vi "resonant.scan.engine_rrMD.vi"() -> ()   [LabVIEW 2012]
doc: "SciScan 1.2 160622"
uses:
  <vilib>/Utility/VariantDataType/Type.ctl
  hyperscope modules/hyperscope subVIs/Timebase and Trigger Routing.ctl
  GFG/GFGnumericGet.vi
  GFG/GFGbooleanGet.vi
  GFG/GFGstringGet.vi
  <vilib>/Utility/error.llb/Error Cluster From Error Code.vi
  <vilib>/rvi/errors/niLvFpgaAdjustHostInterfaceError.vi
  GFG/GFGfpRefGet.vi
  <vilib>/FPGAPlugInAG/Dynamic/niLvFpga_Abort_Dynamic.vi
  <vilib>/FPGAPlugInAG/Dynamic/niLvFpga_Close_Dynamic.vi
  <vilib>/rvi/interface/nirviReadWriteControl/nirviReadWriteControl.xnode
  Custom Controls/FPGA reference typedef for 120MHz code.ctl
  <vilib>/rvi/interface/nirviMethod/nirviMethod.xnode
  <vilib>/rvi/interface/nirviCloseFPGA/nirviCloseFPGA.xnode
  GFG/GFG library.lvlib
  <vilib>/Utility/VariantDataType/VariantType.lvlib
  NiFpgaLv.dll
  <vilib>/rvi/interface/Simulation/niFpgaSimulationCallBeginRW.vi
  <vilib>/FPGAPlugInAG/Dynamic/niLvFpga_ReadFifo_Dynamic.vi
  <vilib>/rvi/errors/niLvFpgaMergeErrorWithErrorCode.vi
panel:
  out "error out 2":errorcluster
  out "error out":errorcluster
  out "x/y":dbl format="%#_6f"
  out "max Elements Remaining":u32
  out "size(s)":i32[](array[numeric])
  out "Elements Remaining":u32
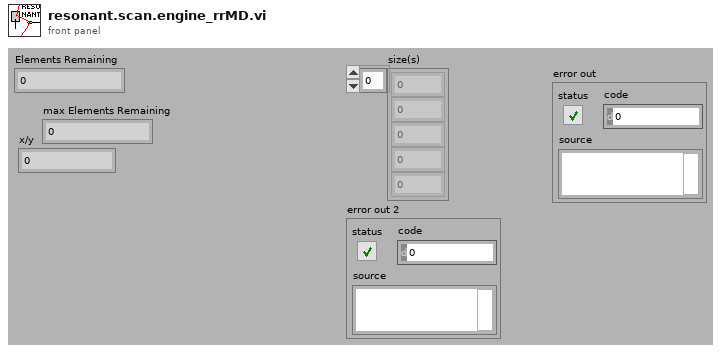
[diagram p1: front panel]
types:
  T1 = typedef "Timebase and Trigger Routing.ctl" = enum16{"Connect", "Disconnect all", "Disconnect Trigger"}
  T2 = enum8{"Enabled", "Disabled", "Disabled and Grayed Out"}
  T3 = typedef "biotfile select.ctl" = enum16{"7962with5751_512px_40Mhz", "7962with5751_512px_50Mhz", "7961with5734_1024px_120Mhz or ext lasersync", "7962with5734_1024px_120Mhz or ext lasersync", "7962with5734_512px_120Mhz or ext lasersync", "7961with5734_512px_120Mhz or ext lasersync", "7962with5751_12kHz_512px_50MHz_4ch", "7962with5751_1536px_2ch_40Mhz", "7962with5751_1536px_2ch_50Mhz", "7962with5751_12kHz_1024px_2ch_50MHz"}
  T4 = typedef "FPGA reference typedef for 120MHz code.ctl" = refnum<k20>
  T5 = cluster{"[0]":bool, "[1]":bool, "[2]":bool, "[3]":bool, "[4]":bool, "[5]":bool, "[6]":bool, "[7]":bool, "[8]":bool}
  T6 = cluster{cluster{"[0]":bool, "[1]":bool, "[2]":bool, "[3]":bool, "[4]":bool, "[5]":bool, "[6]":bool, "[7]":bool, "[8]":bool}, cluster{"[0]":bool, "[1]":bool, "[2]":bool, "[3]":bool, "[4]":bool, "[5]":bool, "[6]":bool, "[7]":bool, "[8]":bool}}
  T7 = cluster{"WaveformChartRef":refnum<vi>, "DigitalRef":refnum<vi>, "ArrayRef":refnum<vi>, "TabControlRef":refnum<vi>, "EnumRef":refnum<vi>, "RingRef":refnum<vi>, "BooleanRef":refnum<vi>, "KnobRef":refnum<vi>, "SlideRef":refnum<vi>, "PathRef":refnum<vi>, "StringRef":refnum<vi>, "ComboBox":refnum<vi>, "WaveformGraphRef":refnum<vi>}
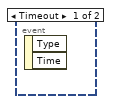
[diagram p5: hidden frame]
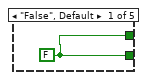
[diagram p6: hidden frame]
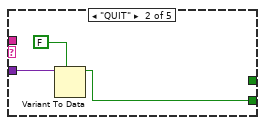
[diagram p7: hidden frame]
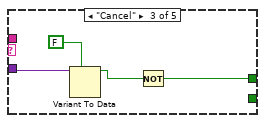
[diagram p8: hidden frame]
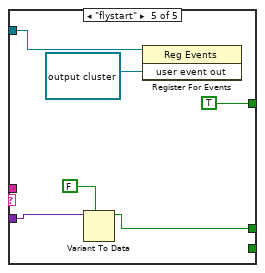
[diagram p10: hidden frame]
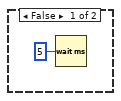
[diagram p11: hidden frame]
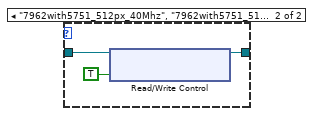
[diagram p12: hidden frame]
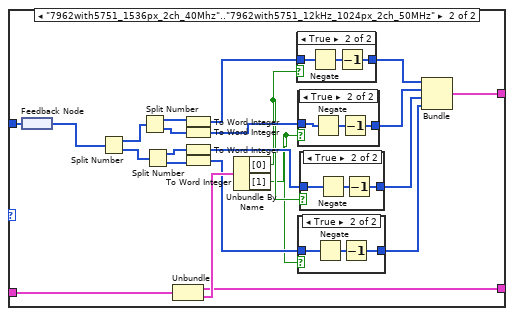
[diagram p20: hidden frame]
diagram:
  n1 = call "GFG_core.vi"() -> ("user event out"=w2:refnum<user-event>)  [unwired: 13 in, 6 out]
  n2 = register-events(w2) -> (reference out=w3:refnum<event-registration>)  [unwired: 2 in, 1 out]
  n3 = while {
    shift-right: [w4] -> _
    shift-left: w3 -> [w11]
    tunnel: w2 -> [w10]
    border: u32 1000000 ("Elements Remaining") -> [_]
    stop <- w12 stop-if-true
    n4 = event shown="[1] <user event out>: User Event" {
      selector: w11 -> [_ w32]
      dyn-events: [_ _] -> w8
      timeout: _ -> [_ _]
      tunnel: [_ w36] -> w13
      tunnel: [_ w35] -> w12
      tunnel: [_ w31] -> w7
      tunnel: [_ w30] -> w6
      event Timeout {
        n5 = event-data() -> ()  [unwired: 1 in, 2 out]
      }
      event User Event {
        n6 = event-data() -> ("Source VI"=w33:string, "Variable Name"=w30:string, "Variant"=w34:variant)  [unwired: 1 in, 4 out]
        n7 = case shown="\"FOCUS\", \"Record\"" w30 {
          tunnel: [w37 _ w41 w49 w54] -> w36
          tunnel: [w37 w38 _ _ _] -> w35
          tunnel: w34 -> [_ w40 w43 w50 w58]
          tunnel: w33 -> [_ _ _ w48 _]
          tunnel: w32 -> [_ _ _ w46 w55]
          tunnel: [_ _ _ TRUE TRUE] -> w31
          frame "False", Default {
            w37 = FALSE ("NewVal")
          }
          frame "QUIT" {
            n8 = Variant To Data(type=FALSE ("NewVal"), Variant=w40) -> (data=w38:bool)  [unwired: 1 in, 1 out]
          }
          frame "Cancel" {
            n9 = Variant To Data(type=FALSE ("NewVal"), Variant=w43) -> (data=w42:bool)  [unwired: 1 in, 1 out]
            n10 = Not(x=w42) -> (.not. x?=w41:bool)
          }
          frame "FOCUS", "Record" {
            n11 = case shown="\"fp button handler_crMD.vi\"" w48 {
              tunnel: w50 -> [_ w52]
              tunnel: [_ w51] -> w49
              frame "False", Default {
              }
              frame "fp button handler_crMD.vi" {
                n12 = Variant To Data(type=FALSE ("NewVal"), Variant=w52) -> (data=w51:bool)  [unwired: 1 in, 1 out]
              }
            }
            n13 = register-events(reference=w46, refnum<user-event> refnum ("user event out")) -> ()  [unwired: 1 in, 2 out]
          }
          frame "flystart" {
            n14 = Variant To Data(type=FALSE ("NewVal"), Variant=w58) -> (data=w54:bool)  [unwired: 1 in, 1 out]
            n15 = register-events(reference=w55, refnum<user-event> refnum ("user event out")) -> ()  [unwired: 1 in, 2 out]
          }
        }
      }
    }
    n16 = case shown="True" w13 {
      tunnel: [_ w120] -> w9
      tunnel: w6 -> [_ w102]
      tunnel: [_ w112] -> w5
      frame False {
        n17 = Wait (ms)(milliseconds to wait=u32 5) -> ()  [unwired: 1 out]
      }
      frame True {
        (unwired) FALSE
        w80 = u64[] [] ("Data")
        n18 = call "GFG_core.vi"("Variable Name in"="flystart" ("Tag in"), "Variant in"=FALSE, "Action"=enum16{"Init", "Set", "Get"}."Set") -> ("error out"=w113:errorcluster)  [unwired: 10 in, 6 out]
        n19 = flat-sequence {
          tunnel: w102 -> [w192]
          tunnel: [w192] -> w61
          tunnel: [w198] -> w101
          tunnel: w61 -> [w198]
          frame #0 {
            n20 = call "GFG_core.vi"("Variable Name in"="scanengine_running", "Variant in"=TRUE, "Action"=enum16{"Init", "Set", "Get"}."Set") -> ()  [unwired: 10 in, 7 out]
          }
          frame #1 {
            n21 = call "GFG_core.vi"("Variable Name in"="flystop", "Variant in"=FALSE ("Boolean"), "Action"=enum16{"Init", "Set", "Get"}."Set") -> ()  [unwired: 10 in, 7 out]
            n22 = call "disable fp elements during scanning.vi"("T for grey out"=TRUE) -> ()  [unwired: 11 in]
            n23 = call "GFG_core.vi"("Variable Name in"="display every n-th frame" ("Tag in"), "Variant in"=2.0 ("Numeric"), "Action"=enum16{"Init", "Set", "Get"}."Set") -> ()  [unwired: 10 in, 7 out]
          }
        }
        n24 = call-poly "GFGpolyGet.vi"("Variable Name in"="frames.p.queue.item" ("Tag in")) -> ("Numeric"=w107:dbl)  [unwired: 8 in, 2 out]
        n25 = call-poly "GFGpolyGet.vi"("error in (no error)"=w113, "Variable Name in"="no..of.frames.to.acquire" ("Tag in")) -> ("Numeric"=w106:dbl)  [unwired: 7 in, 2 out]
        n26 = Divide(x=w106, y=w107) -> (x/y=w108:dbl)
        n27 = flat-sequence {
          tunnel: w94 -> [w150]
          tunnel: w93 -> [w149]
          tunnel: w77 -> [_]
          tunnel: [errorcluster {"status"=FALSE, "code"=0, "source"=""} ("error out")] -> w76
          tunnel: [w153] -> w75
          tunnel: [w152] -> w74
          tunnel: [w151] -> w73
          tunnel: [w148] -> w72
          tunnel: w76 -> [w162]
          tunnel: w75 -> [w161]
          tunnel: w74 -> [w160]
          tunnel: w73 -> [w159]
          tunnel: w72 -> [w158]
          tunnel: [w162] -> w69
          tunnel: [w161] -> w68
          tunnel: [w160] -> w67
          tunnel: [w159] -> w66
          tunnel: [w158] -> w65
          tunnel: [w164] -> w70
          tunnel: [w165] -> w82
          tunnel: [w166] -> w79
          tunnel: [w167] -> w71
          tunnel: [w168] -> w64
          tunnel: w69 -> [w168]
          tunnel: w68 -> [w167]
          tunnel: w67 -> [w166]
          tunnel: w66 -> [w165]
          tunnel: w65 -> [w164]
          frame #0 {
            n28 = call-poly "GFGpolyGet.vi"("Variable Name in"="Hyperscope") -> ("Boolean Value OUT"=w143:bool)  [unwired: 9 in, 1 out]
            n29 = case shown="True" w143 {
              frame False {
              }
              frame True {
                n30 = call-poly "GFGpolyGet.vi"("Variable Name in"="scanner.type") -> ("String"=w146:string)  [unwired: 9 in, 1 out]
                n31 = call "Timebase and Trigger Routing.vi"("Signal Router Action"=Timebase_and_Trigger_Routing."Connect", "System Type"=w146) -> ()  [unwired: 9 in, 1 out]
              }
            }
          }
          frame #1 {
            n32 = call "configure resonance.vi"("x resonant zoom voltage"=w149, "Start Delay (Ticks)"=w150) -> ("bitfile name"=w148:T3, "pixels per frame"=w152:dbl, "FPGA VI Reference Out"=w153:T4, "Actual Depth 3"=w151:u32)  [unwired: 6 in]
          }
          frame #2 {
            n33 = call "GFG_core.vi"("Variable Name in"="shutter" ("Tag in"), "Variant in"=TRUE, "Action"=enum16{"Init", "Set", "Get"}."Set") -> ()  [unwired: 10 in, 7 out]
          }
          frame #3 {
            n34 = Wait (ms)(milliseconds to wait=u32 20) -> ()  [unwired: 1 out]
          }
        }
        n35 = Increment(x=w108) -> (x+1=w103:dbl)
        n36 = call "check focus or flystart.vi"("GFG variable name"=w101) -> ("Focus or flystart?"=w77:bool)  [unwired: 10 in]
        n37 = Round Toward +Infinity(x=w103) -> (ceil(x): smallest int >= x=w105:dbl)
        n38 = Select(t=inf, s=w77, f=w105) -> (s? t:f=w117:dbl)
        n39 = call-poly "GFGpolyGet.vi"("Variable Name in"="Start.Delay" ("Tag in")) -> ("Numeric"=w94:dbl)  [unwired: 8 in, 2 out]
        n40 = call-poly "GFGpolyGet.vi"("Variable Name in"="x.voltage" ("Tag in")) -> ("Numeric"=w93:dbl)  [unwired: 8 in, 2 out]
        n41 = for {
          N: 4 -> [_]
          tunnel: "save.ch." ("Tag in") -> [w175]
          tunnel: [w173] -> w88 mode=indexing
          tunnel: "invert.ch." ("Tag in") -> [w171]
          tunnel: [w169] -> w87 mode=indexing
          i -> [w177]
          n42 = Increment(x=w177) -> (x+1=w176:i32)
          n43 = Number To Decimal String(number=w176) -> (decimal integer string=w170:string)  [unwired: 1 in]
          n44 = Concatenate Strings(w175, w170) -> (w174:string)
          n45 = Concatenate Strings(w171, w170) -> (w172:string)
          n46 = call-poly "GFGpolyGet.vi"("Variable Name in"=w174) -> ("Boolean Value OUT"=w173:bool)  [unwired: 9 in, 1 out]
          n47 = call-poly "GFGpolyGet.vi"("Variable Name in"=w172) -> ("Boolean Value OUT"=w169:bool)  [unwired: 9 in, 1 out]
        }
        n48 = Array To Cluster(array=w88) -> (cluster=w86:T5)
        n49 = Array To Cluster(array=w87) -> (cluster=w85:T5)
        n50 = Boolean To (0,1)(Boolean=w88) -> (0, 1=w91:i16[])
        n51 = Bundle(w86, w85) -> (w84:T6)  [unwired: 1 in]
        n52 = Add Array Elements(numeric array=w91) -> (sum=w90:i16)
        n53 = case shown="Default" w70 {
          tunnel: [w135 w138] -> w63
          tunnel: w71 -> [w134 w137]
          frame Default {
            n54 = xnode "Read/Write Control"("FPGA VI Reference In"=w134, "stop IO config loop"=TRUE, "stop IO config loop"=FALSE) -> ("FPGA VI Reference Out"=w135:T4)  [unwired: 1 in, 1 out]
          }
          frame "7962with5751_512px_40Mhz", "7962with5751_512px_50Mhz", "7962with5751_12kHz_512px_50MHz_4ch".."7962with5751_12kHz_1024px_2ch_50MHz" {
            n55 = xnode "Read/Write Control"("FPGA VI Reference In"=w137, "stop IO config loop"=TRUE) -> ("FPGA VI Reference Out"=w138:T4)  [unwired: 1 in, 1 out]
          }
        }
        n56 = case shown="\"7962with5751_1536px_2ch_40Mhz\"..\"7962with5751_12kHz_1024px_2ch_50MHz\"" w70 {
          tunnel: w79 -> [w139 w141]
          tunnel: [w139 w140] -> w78
          frame Default {
          }
          frame "7962with5751_1536px_2ch_40Mhz".."7962with5751_12kHz_1024px_2ch_50MHz" {
            n57 = Divide(x=w141, y=2.0) -> (x/y=w140:dbl)
          }
        }
        n58 = Initialize Array(i16 0, w107, w90, w79) -> (w81:i16[][][])
        n59 = Obtain Queue(name (unnamed)="resonance raw queue", element data type=w81) -> (queue out=w62:refnum<queue>)  [unwired: 3 in, 2 out]
        n60 = Tick Count (ms)() -> (millisecond timer value=w100:u32)
        n61 = flat-sequence {
          tunnel: w64 -> [_]
          tunnel: w63 -> [w131]
          tunnel: w62 -> [w130]
          frame #0 {
            n62 = call "external trigger warning resonant.vi"("queue ref in"=w130, "FPGA VI Reference In"=w131) -> ()  [unwired: 10 in]
          }
        }
        n63 = while {
          tunnel: [w234] -> w110
          tunnel: w62 -> [w237]
          tunnel: [w236] -> w129
          tunnel: w117 -> [w235]
          tunnel: w64 -> [w228]
          tunnel: w63 -> [w214]
          tunnel: w78 -> [w229]
          tunnel: [w227] -> w124
          tunnel: [w226] -> w122
          tunnel: w77 -> [w207]
          tunnel: w106 -> [w225]
          tunnel: [w202] -> w112
          shift-right: [w203] -> _
          shift-left: w81 -> [w230]
          tunnel: w107 -> [w211]
          tunnel: w107 -> [_]
          border: 0 ("x+y") -> [_]
          tunnel: w82 -> [w218]
          shift-right: [w215] -> _
          shift-left: 0 ("x+y") -> [w216]
          border: w100 -> [_]
          tunnel: w84 -> [w213]
          tunnel: w70 -> [w205]
          border: w80 -> [_]
          border: w80 -> [_]
          i -> [w209]
          stop <- w202 stop-if-true
          n64 = Equal To 0?(x=w209) -> (x = 0?=w201:bool)
          n65 = Increment(x=w209) -> (x+1=w212:i32)
          n66 = Increment(x=w211) -> (x+1=w204:dbl)
          n67 = Select(t=w204, s=w201, f=w211) -> (s? t:f=w210:dbl)
          n68 = case shown="True" w201 {
            frame False {
            }
            frame True {
              n69 = Build Array("Start.Delay" ("Variable Name in"), "ZOOM" ("Variable Name in"), "x.correction" ("Variable Name in")) -> (w238:string[])
              n70 = for {
                tunnel: w238 -> [w242] mode=indexing
                n71 = call-poly "GFGpolyGet.vi"("Variable Name in"=w242) -> ("output cluster"=w245:T7)  [unwired: 9 in, 1 out]
                n72 = Unbundle By Name(w245) -> ("SlideRef"=w243:refnum<vi>)
                n73 = property class="Slide"(reference=w243, "DisabledEnum"=T2."Enabled" ("Disabled")) -> ()  [unwired: 1 in, 2 out]
              }
            }
          }
          n74 = for {
            N: w210 -> [_]
            tunnel: [w283] -> w219
            tunnel: w228 -> [w283]
            tunnel: w229 -> [w253]
            tunnel: w214 -> [w282]
            shift-right: [w280] -> w203
            shift-left: w230 -> [w281]
            tunnel: w211 -> [w279]
            tunnel: w201 -> [w278]
            tunnel: w218 -> [w277]
            shift-right: [w275] -> w215
            shift-left: w216 -> [w276]
            tunnel: w209 -> [w274]
            tunnel: w213 -> [w271]
            tunnel: w201 -> [w270]
            tunnel: w205 -> [w247]
            i -> [w269]
            n75 = xnode "Invoke Method"("FPGA VI Reference In"=w282, "Number of Elements"=w253, "Timeout (ms)"=-1) -> ("error out"=→"error out 2":errorcluster, "Data"=w273:u64[], "Elements Remaining"=w254:u32)  [unwired: 1 in, 1 out]
            "Elements Remaining" <- w254
            n76 = case shown="Default" w247 {
              tunnel: w273 -> [w307 w345]
              tunnel: w271 -> [w306 w344]
              tunnel: [w285 w327] -> w251
              tunnel: [w284 w326] -> w250
              frame Default {
                n77 = feedback #1() -> (w303:u64[])
                n78 = feedback-in #1(w307) -> ()
                n79 = Split Number(x=w303) -> (hi(x)=w304:u32[], lo(x)=w305:u32[])
                n80 = Split Number(x=w304) -> (hi(x)=w301:u16[], lo(x)=w302:u16[])
                n81 = Split Number(x=w305) -> (hi(x)=w300:u16[], lo(x)=w299:u16[])
                n82 = Unbundle(w306) -> (w284:T5, w298:T5)
                n83 = To Word Integer(number=w301) -> (16bit integer=w290:i16[])
                n84 = To Word Integer(number=w302) -> (16bit integer=w292:i16[])
                n85 = To Word Integer(number=w300) -> (16bit integer=w293:i16[])
                n86 = To Word Integer(number=w299) -> (16bit integer=w291:i16[])
                n87 = Unbundle By Name(w298) -> ("[0]"=w297:bool, "[1]"=w296:bool, "[2]"=w295:bool, "[3]"=w294:bool)
                n88 = case shown="True" w297 {
                  tunnel: [w320 w321] -> w289
                  tunnel: w290 -> [w320 w323]
                  frame False {
                  }
                  frame True {
                    n89 = Negate(x=w323) -> (-x=w322:i16[])
                    n90 = Decrement(x=w322) -> (x-1=w321:i16[])
                  }
                }
                n91 = case shown="True" w296 {
                  tunnel: [w316 w317] -> w288
                  tunnel: w292 -> [w316 w319]
                  frame False {
                  }
                  frame True {
                    n92 = Negate(x=w319) -> (-x=w318:i16[])
                    n93 = Decrement(x=w318) -> (x-1=w317:i16[])
                  }
                }
                n94 = case shown="True" w294 {
                  tunnel: [w308 w309] -> w286
                  tunnel: w291 -> [w308 w311]
                  frame False {
                  }
                  frame True {
                    n95 = Negate(x=w311) -> (-x=w310:i16[])
                    n96 = Decrement(x=w310) -> (x-1=w309:i16[])
                  }
                }
                n97 = case shown="True" w295 {
                  tunnel: [w312 w313] -> w287
                  tunnel: w293 -> [w312 w315]
                  frame False {
                  }
                  frame True {
                    n98 = Negate(x=w315) -> (-x=w314:i16[])
                    n99 = Decrement(x=w314) -> (x-1=w313:i16[])
                  }
                }
                n100 = Bundle(w289, w288, w287, w286) -> (w285:cluster{i16[], i16[], i16[], i16[]})  [unwired: 1 in]
              }
              frame "7962with5751_1536px_2ch_40Mhz".."7962with5751_12kHz_1024px_2ch_50MHz" {
                n101 = feedback #2() -> (w341:u64[])
                n102 = feedback-in #2(w345) -> ()
                n103 = Split Number(x=w341) -> (hi(x)=w342:u32[], lo(x)=w343:u32[])
                n104 = Split Number(x=w342) -> (hi(x)=w339:u16[], lo(x)=w340:u16[])
                n105 = Split Number(x=w343) -> (hi(x)=w338:u16[], lo(x)=w337:u16[])
                n106 = Unbundle(w344) -> (w326:T5, w336:T5)
                n107 = To Word Integer(number=w339) -> (16bit integer=w332:i16[])
                n108 = To Word Integer(number=w340) -> (16bit integer=w334:i16[])
                n109 = To Word Integer(number=w338) -> (16bit integer=w335:i16[])
                n110 = To Word Integer(number=w337) -> (16bit integer=w333:i16[])
                n111 = Unbundle By Name(w336) -> ("[0]"=w325:bool, "[1]"=w324:bool)
                n112 = case shown="True" w325 {
                  tunnel: [w358 w359] -> w331
                  tunnel: w332 -> [w358 w361]
                  frame False {
                  }
                  frame True {
                    n113 = Negate(x=w361) -> (-x=w360:i16[])
                    n114 = Decrement(x=w360) -> (x-1=w359:i16[])
                  }
                }
                n115 = case shown="True" w324 {
                  tunnel: [w354 w355] -> w330
                  tunnel: w334 -> [w354 w357]
                  frame False {
                  }
                  frame True {
                    n116 = Negate(x=w357) -> (-x=w356:i16[])
                    n117 = Decrement(x=w356) -> (x-1=w355:i16[])
                  }
                }
                n118 = case shown="True" w324 {
                  tunnel: [w346 w347] -> w328
                  tunnel: w333 -> [w346 w349]
                  frame False {
                  }
                  frame True {
                    n119 = Negate(x=w349) -> (-x=w348:i16[])
                    n120 = Decrement(x=w348) -> (x-1=w347:i16[])
                  }
                }
                n121 = case shown="True" w325 {
                  tunnel: [w350 w351] -> w329
                  tunnel: w335 -> [w350 w353]
                  frame False {
                  }
                  frame True {
                    n122 = Negate(x=w353) -> (-x=w352:i16[])
                    n123 = Decrement(x=w352) -> (x-1=w351:i16[])
                  }
                }
                n124 = Bundle(w331, w330, w329, w328) -> (w327:cluster{i16[], i16[], i16[], i16[]})  [unwired: 1 in]
              }
            }
            n125 = feedback #3() -> (w260:u32)
            n126 = Greater?(x=w254, y=w260) -> (0:w262:bool)
            n127 = Or(x=w262, y=w278) -> (x .or. y?=w259:bool)
            n128 = feedback #4() -> (w248:u32)  [unwired: 1 in]
            n129 = case shown="True" w259 {
              tunnel: w254 -> [_ w460]
              tunnel: [w452 w460] -> w261
              tunnel: w260 -> [w452 _]
              tunnel: w277 -> [_ w459]
              tunnel: [w451 u32 1 ("x")] -> w249
              tunnel: w248 -> [w450 _]
              frame False {
                n130 = Increment(x=w450) -> (x+1=w451:u32)
              }
              frame True {
                n131 = Divide(x=w460, y=w459) -> (x/y=w458:dbl)
                n132 = Multiply(x=w458, y=100.0) -> (x*y=w455:dbl)
                "x/y" <- w455
                n133 = Greater?(x=w455, y=10.0) -> (0:w456:bool)
                n134 = case shown="True" w456 {
                  frame False {
                  }
                  frame True {
                    w463 = "display every n-th frame" ("Tag in")
                    n135 = call-poly "GFGpolyGet.vi"("Variable Name in"=w463) -> ("Numeric"=w462:dbl)  [unwired: 8 in, 2 out]
                    n136 = Increment(x=w462) -> (x+1=w461:dbl)
                    n137 = call "GFG_core.vi"("Variable Name in"=w463, "Variant in"=w461, "Action"=enum16{"Init", "Set", "Get"}."Set") -> ()  [unwired: 10 in, 7 out]
                  }
                }
                "max Elements Remaining" <- w460
              }
            }
            n138 = feedback-in #3(w261) -> ()
            n139 = feedback-in #4(w249) -> ()
            n140 = Less Or Equal?(x=w269, y=0) -> (x <= y?=w256:bool)
            n141 = And(x=w270, y=w256) -> (x .and. y?=w252:bool)
            n142 = Increment(x=w276) -> (x+1=w275:i32)
            n143 = case shown="False" w252 {
              tunnel: w281 -> [w370 w449]
              tunnel: [w369 w449] -> w280
              tunnel: w269 -> [w367 _]
              tunnel: w270 -> [w368 _]
              tunnel: w247 -> [w365 _]
              tunnel: w251 -> [w363 _]
              tunnel: w250 -> [w362 _]
              frame False {
                n144 = Decrement(x=w367) -> (x-1=w364:i32)
                n145 = Select(t=w364, s=w368, f=w367) -> (s? t:f=w366:i32)
                n146 = case shown="\"7962with5751_1536px_2ch_40Mhz\"..\"7962with5751_12kHz_1024px_2ch_50MHz\"" w365 {
                  tunnel: w370 -> [w385 w418]
                  tunnel: [w379 w415] -> w369
                  tunnel: w366 -> [w382 w410]
                  tunnel: w363 -> [w378 w409]
                  tunnel: w362 -> [w373 w404]
                  frame "7962with5751_1536px_2ch_40Mhz".."7962with5751_12kHz_1024px_2ch_50MHz" {
                    n147 = Unbundle(w378) -> (w377:i16[], w374:i16[], w376:i16[], w375:i16[])
                    n148 = Unbundle By Name(w373) -> ("[0]"=w372:bool, "[1]"=w371:bool)
                    n149 = Interleave 1D Arrays(w377, w376) -> (w381:i16[])
                    n150 = Interleave 1D Arrays(w374, w375) -> (w380:i16[])
                    n151 = case shown="True" w372 {
                      tunnel: w385 -> [w393 w399]
                      tunnel: [w393 w398] -> w384
                      tunnel: w382 -> [_ w397]
                      tunnel: w381 -> [_ w396]
                      tunnel: [0 w394] -> w383
                      frame False {
                      }
                      frame True {
                        w395 = 0 ("disabled index (row)")
                        n152 = Increment(x=w395) -> (x+1=w394:i32)
                        n153 = Replace Array Subset(array=w399, new element=w396, index (dim 0)=w397, index (dim 1)=w395) -> (w398:i16[][][])  [unwired: 1 in]
                      }
                    }
                    n154 = case shown="True" w371 {
                      tunnel: w384 -> [w386 w391]
                      tunnel: [w386 w390] -> w379
                      tunnel: w382 -> [_ w389]
                      tunnel: w380 -> [_ w388]
                      tunnel: w383 -> [_ w387]
                      frame False {
                      }
                      frame True {
                        n155 = Replace Array Subset(array=w391, new element=w388, index (dim 0)=w389, index (dim 1)=w387) -> (w390:i16[][][])  [unwired: 1 in]
                      }
                    }
                  }
                  frame Default {
                    n156 = Unbundle By Name(w404) -> ("[0]"=w403:bool, "[1]"=w402:bool, "[2]"=w401:bool, "[3]"=w400:bool)
                    n157 = Unbundle(w409) -> (w408:i16[], w407:i16[], w406:i16[], w405:i16[])
                    n158 = case shown="True" w403 {
                      tunnel: w418 -> [w442 w448]
                      tunnel: [w442 w447] -> w417
                      tunnel: w410 -> [_ w446]
                      tunnel: w408 -> [_ w445]
                      tunnel: [0 w443] -> w413
                      frame False {
                      }
                      frame True {
                        w444 = 0 ("disabled index (row)")
                        n159 = Increment(x=w444) -> (x+1=w443:i32)
                        n160 = Replace Array Subset(array=w448, new element=w445, index (dim 0)=w446, index (dim 1)=w444) -> (w447:i16[][][])  [unwired: 1 in]
                      }
                    }
                    n161 = case shown="True" w402 {
                      tunnel: w417 -> [w434 w440]
                      tunnel: [w434 w439] -> w416
                      tunnel: w410 -> [_ w438]
                      tunnel: w407 -> [_ w437]
                      tunnel: w413 -> [w433 w436]
                      tunnel: [w433 w435] -> w411
                      frame False {
                      }
                      frame True {
                        n162 = Increment(x=w436) -> (x+1=w435:i32)
                        n163 = Replace Array Subset(array=w440, new element=w437, index (dim 0)=w438, index (dim 1)=w436) -> (w439:i16[][][])  [unwired: 1 in]
                      }
                    }
                    n164 = case shown="True" w401 {
                      tunnel: w416 -> [w425 w432]
                      tunnel: w410 -> [_ w431]
                      tunnel: [w425 w430] -> w414
                      tunnel: w406 -> [_ w429]
                      tunnel: [w426 w428] -> w412
                      tunnel: w411 -> [w426 w427]
                      frame False {
                      }
                      frame True {
                        n165 = Increment(x=w427) -> (x+1=w428:i32)
                        n166 = Replace Array Subset(array=w432, new element=w429, index (dim 0)=w431, index (dim 1)=w427) -> (w430:i16[][][])  [unwired: 1 in]
                      }
                    }
                    n167 = case shown="True" w400 {
                      tunnel: [w419 w424] -> w415
                      tunnel: w410 -> [_ w423]
                      tunnel: w414 -> [w419 w422]
                      tunnel: w405 -> [_ w421]
                      tunnel: w412 -> [_ w420]
                      frame False {
                      }
                      frame True {
                        n168 = Replace Array Subset(array=w422, new element=w421, index (dim 0)=w423, index (dim 1)=w420) -> (w424:i16[][][])  [unwired: 1 in]
                      }
                    }
                  }
                }
              }
              frame True {
              }
            }
            n169 = Multiply(x=u32 25, y=w279) -> (x*y=w263:dbl)
            n170 = Equal To 0?(x=w274) -> (x = 0?=w257:bool)
            n171 = feedback #5() -> (w265:i32)
            n172 = Increment(x=w265) -> (x+1=w267:i32)
            n173 = Less Or Equal?(x=w263, y=w267) -> (x <= y?=w266:bool)
            n174 = Or(x=w257, y=w266) -> (x .or. y?=w258:bool)
            n175 = case shown="True" w258 {
              tunnel: w267 -> [w465 _]
              tunnel: [w465 0 ("x+y")] -> w268
              tunnel: w263 -> [_ w471]
              tunnel: w257 -> [_ w467]
              frame False {
              }
              frame True {
                n176 = Not(x=w467) -> (.not. x?=w466:bool)
                n177 = Tick Count (ms)() -> (millisecond timer value=w474:u32)
                n178 = feedback #6() -> (w473:u32)
                n179 = Subtract(x=w474, y=w473) -> (x-y=w472:u32)
                n180 = feedback-in #6(w474) -> ()
                n181 = Divide(x=w472, y=w471) -> (x/y=w470:dbl)
                n182 = Divide(x=1000.0, y=w470) -> (x/y=w468:dbl)
                n183 = case shown="True" w466 {
                  tunnel: w468 -> [_ w478]
                  frame False {
                  }
                  frame True {
                    n184 = call "GFG_core.vi"("Variable Name in"="frames.p.sec", "Variant in"=w478, "Action"=enum16{"Init", "Set", "Get"}."Set") -> ()  [unwired: 10 in, 7 out]
                  }
                }
              }
            }
            n185 = feedback-in #5(w268) -> ()
          }
          n186 = Increment(x=w209) -> (x+1=w208:i32)
          n187 = Multiply(x=w208, y=w211) -> (x*y=w217:dbl)
          n188 = Greater Or Equal?(x=w212, y=w235) -> (x >= y?=w206:bool)
          n189 = flat-sequence {
            tunnel: [w485] -> w223
            tunnel: w219 -> [_]
            tunnel: w217 -> [w492]
            tunnel: w207 -> [w490]
            tunnel: w225 -> [w489]
            tunnel: [w482] -> w222
            tunnel: [w483] -> w221
            tunnel: w206 -> [w479]
            frame #0 {
              n190 = case shown="True" w490 {
                tunnel: w489 -> [_ w501]
                tunnel: w492 -> [w498 w500]
                tunnel: [w498 w499] -> w491
                frame False {
                }
                frame True {
                  n191 = Quotient & Remainder(x=w500, y=w501) -> (x-y*floor(x/y)=w499:dbl)  [unwired: 1 out]
                }
              }
              n192 = call-poly "GFGpolyGet.vi"("Variable Name in"="FOCUS") -> ("Boolean Value OUT"=w485:bool)  [unwired: 9 in, 1 out]
              n193 = call-poly "GFGpolyGet.vi"("Variable Name in"="Record") -> ("Boolean Value OUT"=w486:bool)  [unwired: 9 in, 1 out]
              n194 = call-poly "GFGpolyGet.vi"("Variable Name in"="flystop") -> ("Boolean Value OUT"=w484:bool)  [unwired: 9 in, 1 out]
              n195 = Not(x=w486) -> (.not. x?=w487:bool)
              n196 = And(x=w487, y=w484) -> (x .and. y?=w483:bool)
              n197 = Or(x=w486, y=w485) -> (x .or. y?=w482:bool)
              n198 = Not(x=w479) -> (.not. x?=w480:bool)
              n199 = And(x=w482, y=w480) -> (x .and. y?=w481:bool)
              n200 = case shown="True" w481 {
                tunnel: w491 -> [_ w497]
                frame False {
                }
                frame True {
                  n201 = call "GFG_core.vi"("Variable Name in"="frame.count", "Variant in"=w497, "Action"=enum16{"Init", "Set", "Get"}."Set") -> ()  [unwired: 10 in, 7 out]
                }
              }
            }
          }
          n202 = Array Size(array=w203) -> (size(s)=→"size(s)":i32[])
          n203 = Enqueue Element(queue=w237, element=w203, error in (no error)=w219) -> (queue out=w236:refnum<queue>, error out=w234:errorcluster)  [unwired: 1 in, 1 out]
          n204 = Unbundle By Name(w234) -> ("status"=w232:bool)
          n205 = Not(x=w222) -> (.not. x?=w233:bool)
          n206 = Or(x=w206, y=w233) -> (x .or. y?=w231:bool)
          n207 = Or(x=w232, y=w231) -> (x .or. y?=w224:bool)
          n208 = Or(x=w224, y=w221) -> (x .or. y?=w202:bool)
          n209 = case shown="False" w202 {
            tunnel: w214 -> [w502 w506]
            tunnel: [w502 w505] -> w227
            tunnel: [_ w504] -> w226
            tunnel: w223 -> [_ _]
            frame False {
            }
            frame True {
              n210 = xnode "Invoke Method"("FPGA VI Reference In"=w506) -> ("FPGA VI Reference Out"=w505:T4, "error out"=w504:errorcluster)  [unwired: 1 in]
              n211 = call "GFG_core.vi"("Variable Name in"="shutter" ("Tag in"), "Variant in"=FALSE ("Boolean"), "Action"=enum16{"Init", "Set", "Get"}."Set") -> ()  [unwired: 10 in, 7 out]
            }
          }
        }
        n212 = Release Queue(queue=w129, error in (no error)=w110) -> (error out=w97:errorcluster)  [unwired: 1 in, 2 out]
        n213 = xnode "Invoke Method"("FPGA VI Reference In"=w124, "error in"=w122) -> ("FPGA VI Reference Out"=w123:T4, "error out"=w121:errorcluster)
        n214 = for {
          N: 4 -> [_]
          tunnel: "ao taskref" ("Variable Name in") -> [w185]
          tunnel: w97 -> [_]
          tunnel: [w180] -> w96 mode=indexing
          i -> [w187]
          n215 = Number To Decimal String(number=w187) -> (decimal integer string=w186:string)  [unwired: 1 in]
          n216 = Concatenate Strings(w185, w186) -> (w184:string)
          n217 = call "GFG_core.vi"("Variable Name in"=w184, "Action"=enum16{"Init", "Set", "Get"}."Get") -> ("Variant Out"=w182:variant, "error out"=w183:errorcluster)  [unwired: 11 in, 5 out]
          n218 = Variant To Data(error in=w183, type=refnum<k21> refnum ("task out"), Variant=w182) -> (data=w179:refnum<k21>, error out=w178:errorcluster)
          n219 = call <vilib>:"DAQmx Clear Task.vi"("task in"=w179, "error in"=w178) -> ("error out"=w180:errorcluster)  [unwired: 13 in]
        }
        n220 = xnode "Close FPGA VI Reference"("FPGA VI Reference In"=w123) -> ("error out"=w120:errorcluster)  [unwired: 1 in]
        n221 = Merge Errors(w96, w121) -> (→"error out":errorcluster)
      }
    }
    n222 = case shown="True" w7 {
      tunnel: w10 -> [_ w29]
      tunnel: w9 -> [_ _]
      tunnel: [w26 w28] -> w4
      tunnel: w8 -> [w26 w27]
      frame False {
      }
      frame True {
        n223 = register-events(reference=w27, w29) -> (reference out=w28:refnum<event-registration>)  [unwired: 1 in, 1 out]
      }
    }
    n224 = case shown="True" w5 {
      tunnel: w4 -> [_ _]
      frame False {
      }
      frame True {
        n225 = flat-sequence {
          frame #0 {
            n226 = call "reset FPGA DO.vi"() -> ()  [unwired: 12 in]
          }
          frame #1 {
            n227 = call "reset AO.vi"() -> ()  [unwired: 12 in]
          }
          frame #2 {
            n228 = call-poly "GFGpolyGet.vi"("Variable Name in"="Hyperscope") -> ("Boolean Value OUT"=w19:bool)  [unwired: 9 in, 1 out]
            n229 = case shown="True" w19 {
              frame False {
              }
              frame True {
                n230 = call-poly "GFGpolyGet.vi"("Variable Name in"="scanner.type") -> ("String"=w21:string)  [unwired: 9 in, 1 out]
                n231 = call "Timebase and Trigger Routing.vi"("Signal Router Action"=Timebase_and_Trigger_Routing."Disconnect all", "System Type"=w21) -> ()  [unwired: 9 in, 1 out]
              }
            }
          }
          frame #3 {
            n232 = call "GFG_core.vi"("Variable Name in"="scanengine_running", "Variant in"=FALSE, "Action"=enum16{"Init", "Set", "Get"}."Set") -> ()  [unwired: 10 in, 7 out]
          }
        }
        n233 = call "disable fp elements during scanning.vi"("T for grey out"=FALSE) -> ()  [unwired: 11 in]
        n234 = Get Date/Time In Seconds() -> (seconds since 1Jan1904=w15:timestamp)
        n235 = call "GFG_core.vi"("Variable Name in"="resonant.scan.engine_MD.completed", "Variant in"=w15, "Action"=enum16{"Init", "Set", "Get"}."Set") -> ()  [unwired: 10 in, 7 out]
      }
    }
  }
